vi "enqueueForce.vi"(8 "error in (no error)":errorcluster, 10 "Stop":bool, 11 "RawBits":u8[](array[numeric])) -> (0 "error out":errorcluster)   [LabVIEW 2017, in "externalAquisition.lvlib"]
uses:
  externalAquisition.lvlib
  TypeDefs/QueueCommands.ctl
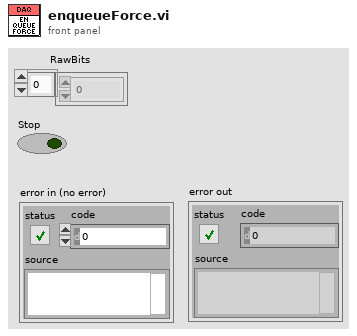
[diagram p1: front panel]
types:
  T1 = typedef "externalAquisition.lvlib/QueueCommands.ctl" = enum16{"get", "set"}
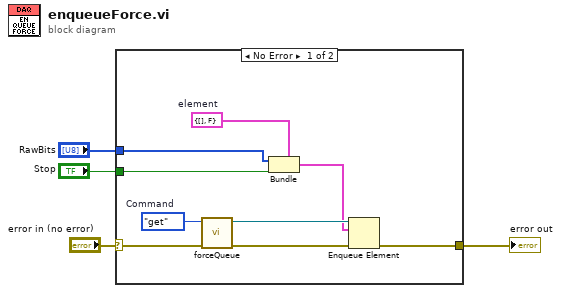
[diagram p0: block diagram]
diagram:
  n1 = case shown="No Error" "error in (no error)" {
    selector: "error in (no error)" -> [w13 w14]
    tunnel: [w5 w14] -> w3
    tunnel: "Stop" -> [w7 _]
    tunnel: "RawBits" -> [w6 _]
    frame No Error {
      w9 = cluster{u8[], "Stop":bool} {[], "Stop"=FALSE}  # element
      w10 = QueueCommands."get"  # Command
      n2 = call "forceQueue.vi"("error in (no error)"=w13, "Command"=w10) -> ("error out"=w12:errorcluster, "queue out"=w11:refnum<queue>)  [unwired: 8 in]
      n3 = Bundle(cluster=w9, w6, "Stop"=w7) -> (w8:cluster{u8[], "Stop":bool})
      n4 = Enqueue Element(queue=w11, element=w8, error in (no error)=w12) -> (error out=w5:errorcluster)  [unwired: 1 in, 2 out]
    }
    frame Error {
    }
  }
  "error out" <- w3
